vi "Averager Compute.vi"(8 "error in (no error)":errorcluster, 10 "Data":dbl[](array[numeric]), 11 "Standard RMS in":refnum<class "Standard RMS.lvclass">) -> (0 "error out":errorcluster, 3 "Standard RMS out":refnum<class "Standard RMS.lvclass">)   [LabVIEW 2018, in "Standard RMS.lvclass"]
uses:
  Standard RMS.lvclass
  C:/Users/aaron.jencks/Documents/GitHub/emerson_seed_object_detection/LabVIEW/Projects/Paul's Video Viewer/Classes/Averager/Averager.lvclass
  <vilib>/Analysis/5stat.llb/RMS (DBL).vi
  Standard Averager/Standard Averager.lvclass
  <vilib>/Analysis/NI_AALPro.lvlib
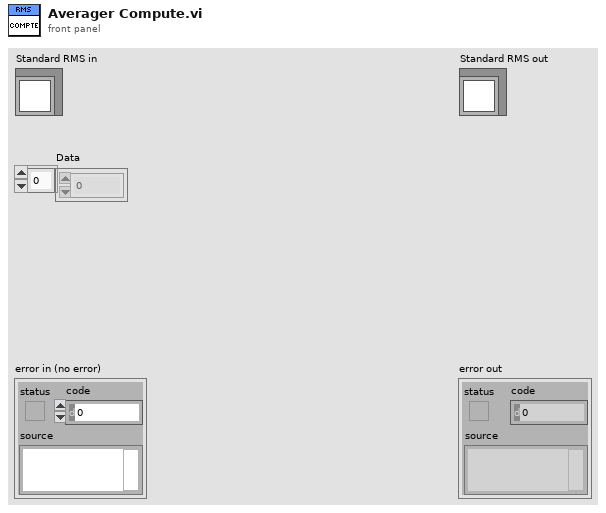
[diagram p1: front panel]
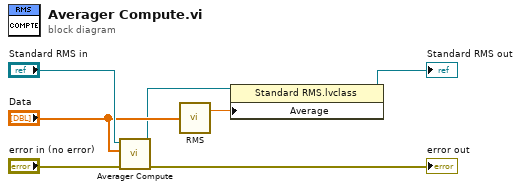
[diagram p0: block diagram]
diagram:
  n1 = call-parent "Averager Compute.vi"("error in (no error)"="error in (no error)", "Data"="Data", "Standard Averager in"="Standard RMS in") -> ("error out"=→"error out":errorcluster, "Standard Averager out"=w3:refnum<class "Standard RMS.lvclass">)  [unwired: 7 in]
  n2 = call-poly <vilib>:"RMS.vi"("X"="Data") -> ("rms value"=w2:dbl)  [unwired: 1 out]
  n3 = property class="Standard RMS.lvclass"(reference=w3, "Average"=w2) -> (reference out=→"Standard RMS out":refnum<class "Standard RMS.lvclass">)  [unwired: 1 in, 1 out]
